vi "Log.vi"(8 "error in":errorcluster, 11 "File Path Control":path) -> (0 "error out":errorcluster, 3 "String 2":string)   [LabVIEW 2014]
uses:
  StopForLog.vi
panel:
  in  "stop":bool
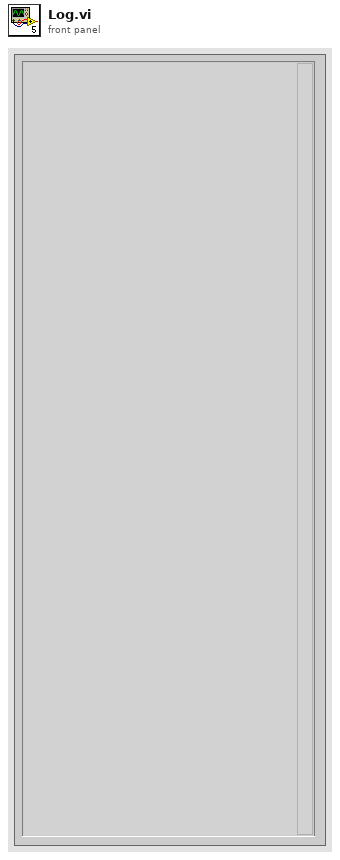
[diagram p1: front panel]
types:
  T1 = enum16{"open", "replace", "create", "open or create", "replace or create", "replace or create with confirmation"}
  T2 = enum32{"Invalid", "Standard", "Closed", "Hidden", "Minimized", "Maximized"}
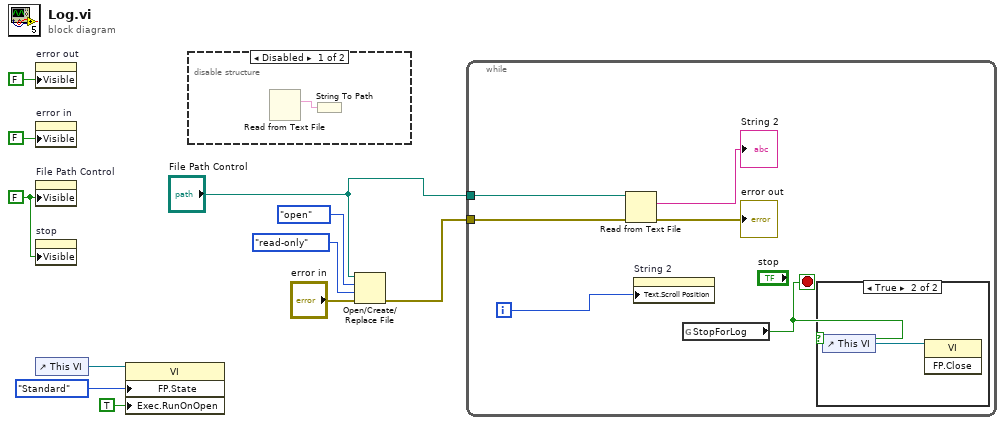
[diagram p0: block diagram]
diagram:
  w8 = FALSE ("Visible")
  n1 = property on="error out" class="Clust (strict)"("Visible"=FALSE) -> ()  [unwired: 2 in, 2 out]
  n2 = property on="error in" class="Clust (strict)"("Visible"=FALSE) -> ()  [unwired: 2 in, 2 out]
  n3 = property on="File Path Control" class="Path"("Visible"=w8) -> ()  [unwired: 2 in, 2 out]
  n4 = property on="stop" class="Bool"("Visible"=w8) -> ()  [unwired: 2 in, 2 out]
  n5 = control-ref of="This VI"() -> (w10:refnum<vi>)
  n6 = property class="VI"(reference=w10, "FP.State"=T2."Standard" ("Front Panel Window:State"), "Exec.RunOnOpen"=TRUE ("Execution:Run When Opened")) -> ()  [unwired: 1 in, 2 out]
  n7 = disable-structure shown="Disabled" {
    frame Disabled {
      n8 = Read from Text File() -> (text=w12:string)  [unwired: 4 in, 3 out]
      n9 = String To Path(string=w12) -> ()  [unwired: 1 out]
    }
    frame Enabled {
    }
  }
  n10 = Open/Create/Replace File(file path (use dialog)="File Path Control", error in="error in", operation (0:open)=T1."open", access (0:read/write)=enum16{"read/write", "read-only", "write-only"}."read-only") -> (error out=w2:errorcluster)  [unwired: 2 in, 2 out]
  n11 = while {
    tunnel: "File Path Control" -> [w14]
    tunnel: w2 -> [w15]
    i -> [w16]
    stop <- w13 stop-if-true
    n12 = Read from Text File(file (use dialog)=w14, error in=w15) -> (text=→"String 2":string, error out=→"error out":errorcluster)  [unwired: 2 in, 2 out]
    n13 = property on="String 2" class="Str"("Text.Scroll Position"=w16) -> ()  [unwired: 2 in, 2 out]
    n14 = global read "StopForLog.vi" "StopForLog"() -> (w13:bool)
    n15 = case shown="True" w13 {
      frame False {
      }
      frame True {
        n16 = control-ref of="This VI"() -> (w19:refnum<vi>)
        n17 = invoke class="VI" method="FP.Close"(reference=w19) -> ()  [unwired: 2 in, 3 out]
      }
    }
  }
